vi "Start Button Pressed.vi"(8 "error in (no error)":errorcluster, 10 "Selected Steps":T1[](array[typedef]), 11 "Car Wash Controller in":refnum<class "Car Wash Controller.lvclass">) -> (0 "error out":errorcluster, 3 "Car Wash Controller out":refnum<class "Car Wash Controller.lvclass">)   [LabVIEW 2012, in "Car Wash Controller.lvlib" / "Car Wash Controller.lvclass"]
uses:
  Car Wash Controller.lvclass
  Car Wash Controller State.ctl
  Wash Step.ctl
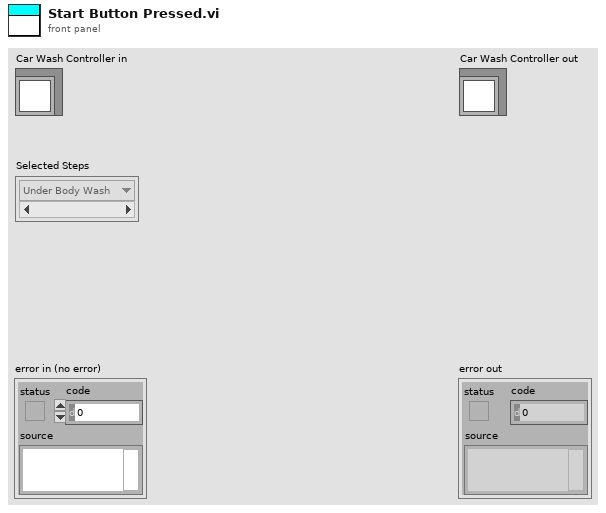
[diagram p1: front panel]
types:
  T1 = typedef "Car Wash Controller.lvlib/Car Wash Controller.lvclass/Wash Step.ctl" = enum16{"Under Body Wash", "Bug Remover", "Pre-Soak", "High Pressure Wash", "Low Pressure Wax", "Spot Free Rince", "Tire Shine Foam", "Air Dry"}
  T2 = typedef "Car Wash Controller.lvlib/Car Wash Controller.lvclass/Car Wash Controller State.ctl" = enum16{"Initial State", "Wait For Start State", "Start State", "Wait For Vehicle Position State", "Wash Step Execution State", "Wash Step / Cycle Completion State", "Wash Exit State", "Wash Abort / Terminate State"}
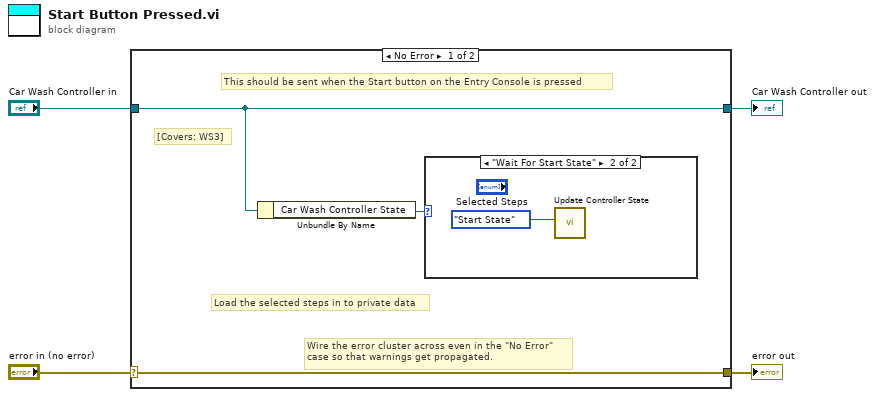
[diagram p0: block diagram]
diagram:
  n1 = case shown="No Error" "error in (no error)" {
    selector: "error in (no error)" -> [w7 w10]
    tunnel: [w7 w10] -> w3
    tunnel: [w6 w9] -> w1
    tunnel: "Car Wash Controller in" -> [w6 w9]
    frame No Error {
      # "Load the selected steps in to private data"
      # "[Covers: WS3]"
      # "This should be sent when the Start button on the Entry Console is pressed"
      # "Wire the error cluster across even in the \"No Error\"\ncase so that warnings get propagated."
      n2 = Unbundle By Name(w6) -> ("Car Wash Controller State"=w5:T2)
      n3 = case shown="\"Wait For Start State\"" w5 {
        frame "Initial State", Default {
        }
        frame "Wait For Start State" {
          n4 = call "Update Controller State.vi"("Car Wash Controller State"=Car_Wash_Controller_State."Start State") -> ()  [unwired: 9 in, 2 out]
        }
      }
    }
    frame Error {
    }
  }
  "error out" <- w3
  "Car Wash Controller out" <- w1
